vi "AddPanel.vi"(8 "error in":errorcluster caption="错误输入（无错误）", 10 "Vi Alias":string, 11 "PanelRootNode 输入":refnum<class "PanelRootNode.lvclass"> caption="DNL_LabVIEW Object in") -> (0 "error out":errorcluster caption="错误输出", 3 "PanelRootNode 输出":refnum<class "PanelRootNode.lvclass"> caption="DNL_LabVIEW Object out")   [LabVIEW 2016, in "PanelRootNode.lvclass"]
uses:
  PanelRootNode.lvclass
  PanelDataNode/Split Mode.ctl
  PanelDataNode/PanelDataNode.lvclass
  C:/Users/CL/Desktop/ZcDAQprj0811/ZcDAQprj/Modules/DAQ-Display/PanelSplitToolkit/PanelObject/PanelObject.lvclass
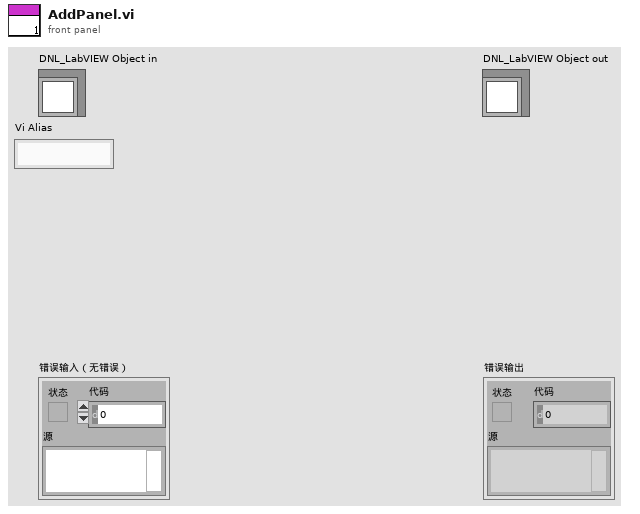
[diagram p1: front panel]
types:
  T1 = typedef "PanelDataNode.lvclass/Split Mode.ctl" = enum16{"Horizontal(up)", "Vertical(left)", "Horizontal(down)", "Vertical(right)"}
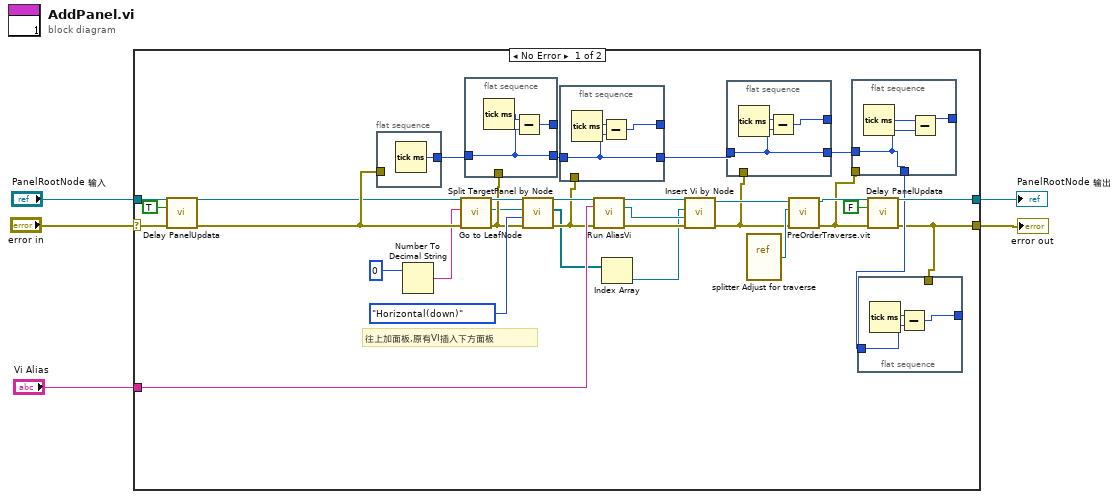
[diagram p0: block diagram]
diagram:
  n1 = case shown="No Error" "error in" {
    selector: "error in" -> [w30 w55]
    tunnel: [w14 w55] -> w4
    tunnel: [w35 w54] -> w2
    tunnel: "PanelRootNode 输入" -> [w32 w54]
    tunnel: "Vi Alias" -> [w37 _]
    frame No Error {
      # "往上加面板,原有VI插入下方面板"
      n2 = call "Delay PanelUpdata.vi"("error in"=w30, "延迟前面板更新"=TRUE, "PanelRootNode 输入"=w32) -> ("error out"=w33:errorcluster, "PanelRootNode 输出"=w31:refnum<class "PanelRootNode.lvclass">)  [unwired: 7 in]
      n3 = flat-sequence {
        tunnel: [w53] -> w22
        tunnel: w33 -> [_]
        frame #0 {
          n4 = Tick Count (ms)() -> (millisecond timer value=w53:u32)
        }
      }
      n5 = Number To Decimal String(number=0) -> (decimal integer string=w28:string)  [unwired: 1 in]
      n6 = call-dynamic "Go to LeafNode.vi"("error in"=w33, "LeafNumber"=w28, "PanelRootNode 输入"=w31) -> ("error out"=w20:errorcluster, "Node*"=w8:refnum<data-value>, "PanelRootNode 输出"=w26:refnum<class "PanelRootNode.lvclass">)  [unwired: 5 in, 1 out]
      n7 = flat-sequence {
        tunnel: [w51] -> w21
        tunnel: w22 -> [w51]
        tunnel: w20 -> [_]
        tunnel: [w50] -> _
        frame #0 {
          n8 = Tick Count (ms)() -> (millisecond timer value=w52:u32)
          n9 = Subtract(x=w52, y=w51) -> (x-y=w50:u32)
        }
      }
      n10 = call-dynamic "Split TargetPanel by Node.vi"("error in"=w20, "Split Mode"=Split_Mode."Horizontal(down)", "Node*"=w8, "PanelRootNode 输入"=w26) -> ("error out"=w19:errorcluster, "ChildDataNode[]"=w7:refnum<data-value>[], "PanelRootNode 输出"=w36:refnum<class "PanelRootNode.lvclass">)  [unwired: 5 in]
      n11 = flat-sequence {
        tunnel: w21 -> [w47]
        tunnel: w19 -> [_]
        tunnel: [w48] -> _
        tunnel: [w47] -> w18
        frame #0 {
          n12 = Tick Count (ms)() -> (millisecond timer value=w49:u32)
          n13 = Subtract(x=w49, y=w47) -> (x-y=w48:u32)
        }
      }
      n14 = call-dynamic "Run AliasVi.vi"("error in (no error)"=w19, "Vi Alias"=w37, "PanelDataNode 输入"=w36) -> ("error out"=w11:errorcluster, "VI*"=w9:refnum<vi>, "PanelDataNode 输出"=w13:refnum<class "PanelRootNode.lvclass">)  [unwired: 6 in]
      n15 = Index Array(array=w7) -> (element=w6:refnum<data-value>)  [unwired: 1 in]
      n16 = call-dynamic "Insert Vi by Node.vi"("error in"=w11, "dynamic VI*"=w9, "Node*"=w6, "PanelRootNode 输入"=w13) -> ("error out"=w10:errorcluster, "PanelRootNode 输出"=w12:refnum<class "PanelRootNode.lvclass">)  [unwired: 6 in]
      n17 = flat-sequence {
        tunnel: w18 -> [w44]
        tunnel: [w45] -> _
        tunnel: w10 -> [_]
        tunnel: [w44] -> w17
        frame #0 {
          n18 = Tick Count (ms)() -> (millisecond timer value=w46:u32)
          n19 = Subtract(x=w46, y=w44) -> (x-y=w45:u32)
        }
      }
      n20 = vi-ref "splitter Adjust for traverse.vi"() -> (w24:refnum<vi>)
      n21 = call-dynamic "PreOrderTraverse.vit"("error in"=w10, "vi reference"=w24, "PanelLinkNode 输入"=w12) -> ("error out"=w16:errorcluster, "PanelLinkNode 输出"=w25:refnum<class "PanelRootNode.lvclass">)  [unwired: 5 in, 2 out]
      n22 = flat-sequence {
        tunnel: w17 -> [w41]
        tunnel: [w42] -> _
        tunnel: w16 -> [_]
        tunnel: [w41] -> w15
        frame #0 {
          n23 = Tick Count (ms)() -> (millisecond timer value=w43:u32)
          n24 = Subtract(x=w43, y=w41) -> (x-y=w42:u32)
        }
      }
      n25 = flat-sequence {
        tunnel: w15 -> [w39]
        tunnel: [w38] -> _
        tunnel: w14 -> [_]
        frame #0 {
          n26 = Tick Count (ms)() -> (millisecond timer value=w40:u32)
          n27 = Subtract(x=w40, y=w39) -> (x-y=w38:u32)
        }
      }
      n28 = call "Delay PanelUpdata.vi"("error in"=w16, "延迟前面板更新"=FALSE, "PanelRootNode 输入"=w25) -> ("error out"=w14:errorcluster, "PanelRootNode 输出"=w35:refnum<class "PanelRootNode.lvclass">)  [unwired: 7 in]
    }
    frame Error {
    }
  }
  "error out" <- w4
  "PanelRootNode 输出" <- w2
